vi "DistanceSensorCrtl.vi"(8 "error in (no error)":errorcluster, 10 "Control Option":enum16{"SetLock", "UnSetLock", "Read"}(ring)=enum."UnSetLock", 11 "VISA resource name":refnum<visa-resource-name>="COM4") -> (0 "error out":errorcluster, 1 "Distance(mm)":dbl, 2 "Result":string, 3 "VISA resource name out":refnum<visa-resource-name>)   [LabVIEW 2019]
uses:
  <vilib>/Instr/_visa.llb/VISA Configure Serial Port (Instr).vi
panel:
  in  "flow control":u16(ring) items=["None"=0, "XON/XOFF"=1, "RTS/CTS"=2, "DTR/DSR"=4]
  in  "stop bits":u16(ring)=10 items=["1"=10, "1.5"=15, "2.0"=20]
  in  "parity":u16(ring)=2 items=["None", "Odd", "Even", "Mark", "Space"]
  in  "data bits":u16=8 min=5 max=8 step=1
  in  "baud rate":u32=1500000
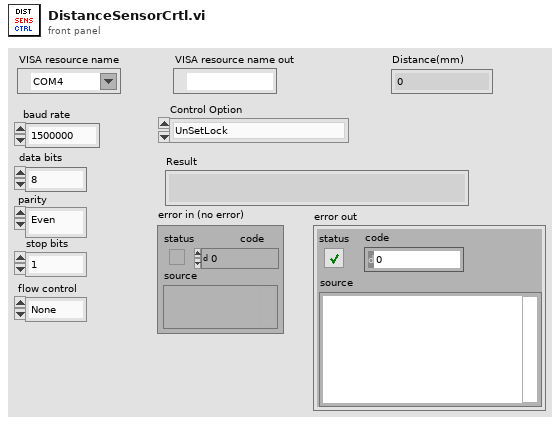
[diagram p1: front panel]
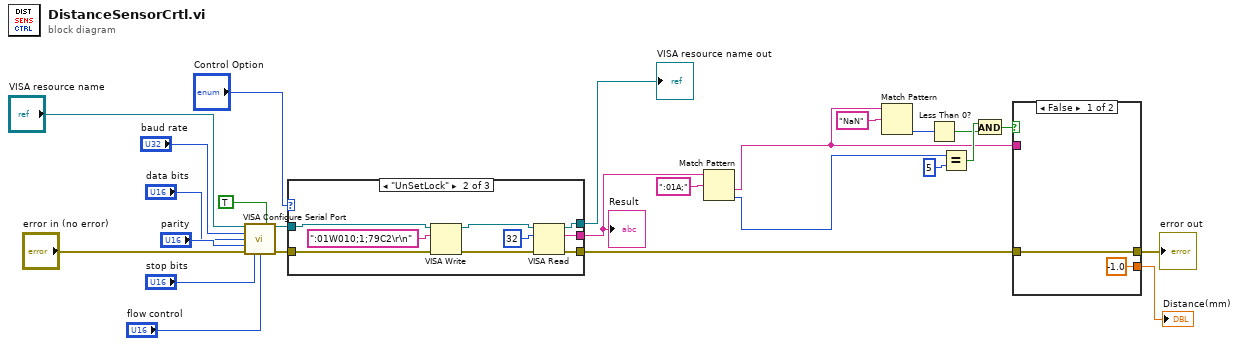
[diagram p0: block diagram]
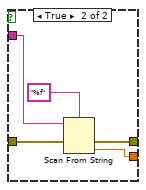
[diagram p2: hidden frame]
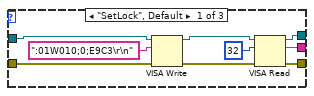
[diagram p3: hidden frame]
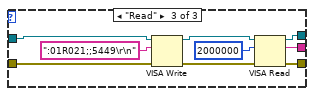
[diagram p4: hidden frame]
diagram:
  n1 = call-poly "VISA Configure Serial Port"("VISA resource name"="VISA resource name", "Enable Termination\nChar (T)"=TRUE, "baud rate (9600)"="baud rate", "data bits (8)"="data bits", "parity (0:none)"="parity", "error in (no error)"="error in (no error)", "stop bits (10: 1 bit)"="stop bits", "flow control (0:none)"="flow control") -> ("VISA resource name out"=w16:refnum<visa-resource-name>, "error out"=w19:errorcluster)  [unwired: 6 in]
  n2 = case shown="\"UnSetLock\"" "Control Option" {
    tunnel: [w30 w42 w47] -> w13
    tunnel: w16 -> [w29 w40 w51]
    tunnel: w19 -> [w28 w39 w52]
    tunnel: [w27 w37 w45] -> w3
    tunnel: [w26 w36 w44] -> w14
    frame "SetLock", Default {
      n3 = VISA Write(VISA resource name=w29, write buffer=":01W010;0;E9C3\r\n", error in (no error)=w28) -> (VISA resource name out=w32:refnum<visa-resource-name>, error out=w31:errorcluster)  [unwired: 1 out]
      n4 = VISA Read(VISA resource name=w32, byte count=u32 32, error in (no error)=w31) -> (VISA resource name out=w26:refnum<visa-resource-name>, read buffer=w30:string, error out=w27:errorcluster)  [unwired: 1 out]
    }
    frame "UnSetLock" {
      n5 = VISA Write(VISA resource name=w40, write buffer=":01W010;1;79C2\r\n", error in (no error)=w39) -> (VISA resource name out=w41:refnum<visa-resource-name>, error out=w35:errorcluster)  [unwired: 1 out]
      n6 = VISA Read(VISA resource name=w41, byte count=u32 32, error in (no error)=w35) -> (VISA resource name out=w36:refnum<visa-resource-name>, read buffer=w42:string, error out=w37:errorcluster)  [unwired: 1 out]
    }
    frame "Read" {
      n7 = VISA Write(VISA resource name=w51, write buffer=":01R021;;5449\r\n" ("Command"), error in (no error)=w52) -> (VISA resource name out=w49:refnum<visa-resource-name>, error out=w48:errorcluster)  [unwired: 1 out]
      n8 = VISA Read(VISA resource name=w49, byte count=u32 2000000, error in (no error)=w48) -> (VISA resource name out=w44:refnum<visa-resource-name>, read buffer=w47:string, error out=w45:errorcluster)  [unwired: 1 out]
    }
  }
  "Result" <- w13
  "VISA resource name out" <- w14
  n9 = Match Pattern(string=w13, regular expression=":01A;") -> (after substring=w4:string, offset past match=w11:i32)  [unwired: 1 in, 2 out]
  n10 = Match Pattern(string=w4, regular expression="NaN") -> (offset past match=w8:i32)  [unwired: 1 in, 3 out]
  n11 = Less Than 0?(x=w8) -> (x < 0?=w6:bool)
  n12 = Equal?(x=w11, y=5) -> (x = y?=w7:bool)
  n13 = And(x=w7, y=w6) -> (x .and. y?=w5:bool)
  n14 = case shown="False" w5 {
    tunnel: w4 -> [_ w59]
    tunnel: w3 -> [w53 w58]
    tunnel: [-1.0 w56] -> w2
    tunnel: [w53 w55] -> w1
    frame False {
    }
    frame True {
      n15 = Scan From String(format string="%f", input string=w59, error in=w58) -> (error out=w55:errorcluster, output 1=w56:dbl)  [unwired: 2 in, 2 out]
    }
  }
  "error out" <- w1
  "Distance(mm)" <- w2
